vi "Dynamic Dispatch Method.vi"(8 "error in (no error)":errorcluster, 11 "class string in":refnum<class "Parent.lvclass">) -> (0 "error out":errorcluster, 2 "String Data":string, 3 "class string out":refnum<class "Parent.lvclass">)   [LabVIEW 2023, in "Parent.lvclass"]
doc: "This is a dynamic dispatch member VI of Parent.lvclass. Use this VI as a VI under test for the Dynamic Dispatch Method.lvtest test."
uses:
  Parent.lvclass
  Parent.lvclass/Parent.ctl
panel:
  # "Overview: This is a dynamic dispatch member VI of Parent.lvclass. Use this VI as a VI under test for the Dynamic Dispatch Method.lvtest test. \nRequirements: LabVIEW Full Development System, Unit Test Framework Toolkit"
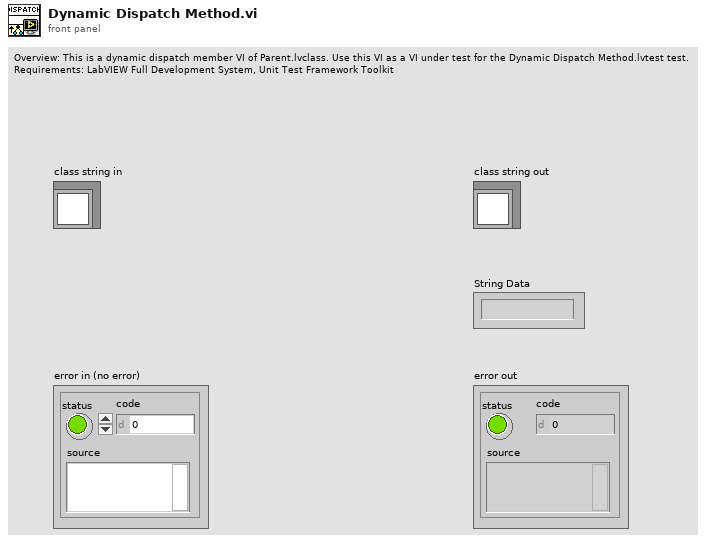
[diagram p1: front panel]
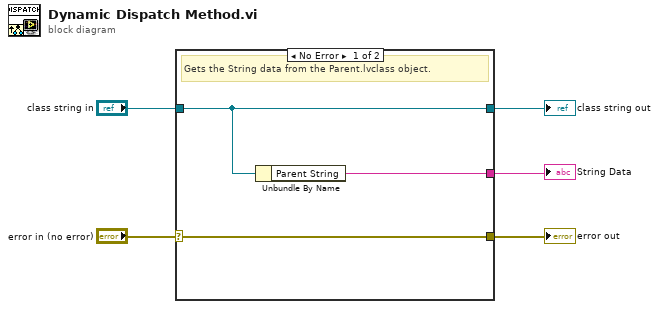
[diagram p0: block diagram]
diagram:
  n1 = case shown="No Error" "error in (no error)" {
    selector: "error in (no error)" -> [w8 w10]
    tunnel: [w8 w10] -> w4
    tunnel: [w7 w9] -> w2
    tunnel: "class string in" -> [w7 w9]
    tunnel: [w6 _] -> w1
    frame No Error {
      # "Gets the String data from the Parent.lvclass object."
      n2 = Unbundle By Name(w7) -> ("Parent String"=w6:string)
    }
    frame Error {
    }
  }
  "error out" <- w4
  "class string out" <- w2
  "String Data" <- w1
